vi "Mark_SetBEMark.vi"(8 "error in (no error)":errorcluster, 9 "End":i32[](array[numeric]), 10 "Begin":i32[](array[numeric]), 11 "CarexData In":refnum<class "ExpData.lvclass">) -> (0 "error out":errorcluster, 3 "CarexData Out":refnum<class "ExpData.lvclass">)   [LabVIEW 2016, in "ExpData.lvclass"]
uses:
  ExpData.lvclass
  ExpData.lvclass/ExpData.ctl
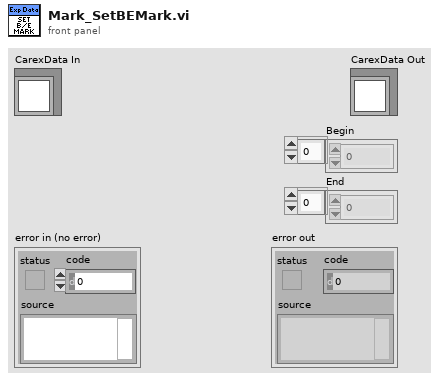
[diagram p1: front panel]
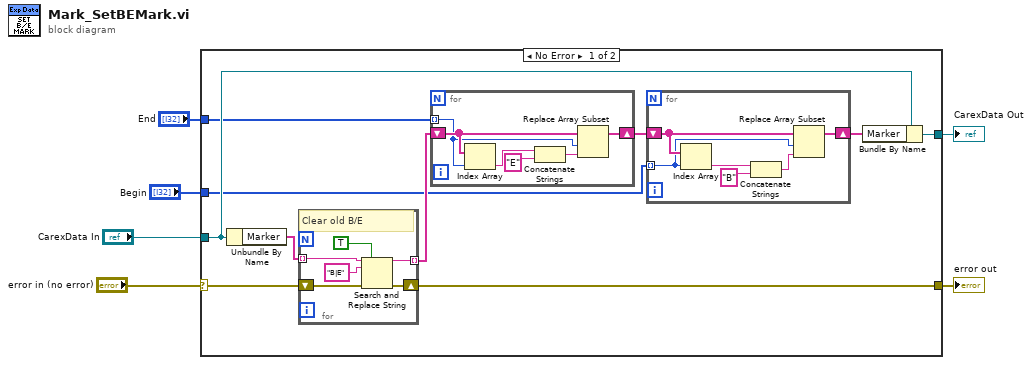
[diagram p0: block diagram]
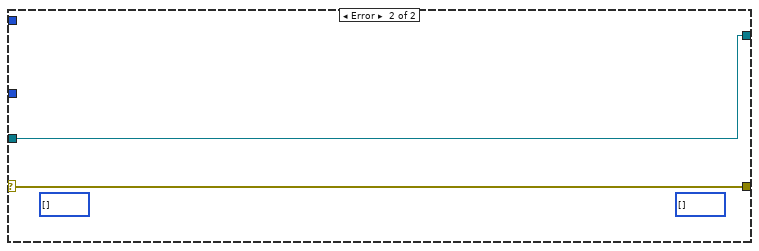
[diagram p2: hidden frame]
diagram:
  n1 = case shown="No Error" "error in (no error)" {
    selector: "error in (no error)" -> [w9 w36]
    tunnel: [w14 w36] -> w1
    tunnel: "CarexData In" -> [w10 w35]
    tunnel: "End" -> [w7 _]
    tunnel: [w12 w35] -> w2
    tunnel: "Begin" -> [w8 _]
    frame No Error {
      n2 = Unbundle By Name(w10) -> ("Marker"=w11:string[])
      n3 = for {
        tunnel: w11 -> [w22] mode=indexing
        tunnel: [w20] -> w15 mode=indexing
        shift-right: [w17] -> w14
        shift-left: w9 -> [w18]
        # "Clear old B/E"
        n4 = Search and Replace String(replace all?=TRUE ("replace all? (F)"), input string=w22, search string="B|E", error in=w18) -> (result string=w20:string, error out=w17:errorcluster)  [unwired: 4 in, 2 out]
      }
      n5 = for {
        tunnel: w7 -> [w32] mode=indexing
        shift-right: [w34] -> w16
        shift-left: w15 -> [w33]
        n6 = Index Array(array=w33, index=w32) -> (element=w30:string)
        n7 = Concatenate Strings(w30, "E" ("new element/subarray")) -> (w31:string)
        n8 = Replace Array Subset(array=w33, new element=w31, index=w32) -> (w34:string[])
      }
      n9 = for {
        tunnel: w8 -> [w26] mode=indexing
        shift-right: [w28] -> w13
        shift-left: w16 -> [w27]
        n10 = Index Array(array=w27, index=w26) -> (element=w24:string)
        n11 = Concatenate Strings(w24, "B" ("new element/subarray")) -> (w25:string)
        n12 = Replace Array Subset(array=w27, new element=w25, index=w26) -> (w28:string[])
      }
      n13 = Bundle By Name(cluster=w10, "Marker"=w13) -> (w12:refnum<class "ExpData.lvclass">)
    }
    frame Error {
      (unwired) i32[] []
      (unwired) i32[] []
    }
  }
  "CarexData Out" <- w2
  "error out" <- w1
